vi "DG535.set input impedance.vi"(0 "i ref in":refnum<vi>, 7 "input impedance":bool, 11 "error in (no error)":errorcluster) -> (4 "i ref out":refnum<vi>, 15 "error out":errorcluster)   [LabVIEW 2014, in "DG535.lvlib"]
doc: "2 to 32766.\nThis command is used to specify the number of pulses, which will be in each burst of pulses when in the burst mode."
uses:
  DG535.lvlib
panel:
  # "50 Ohms"
  # "High Z"
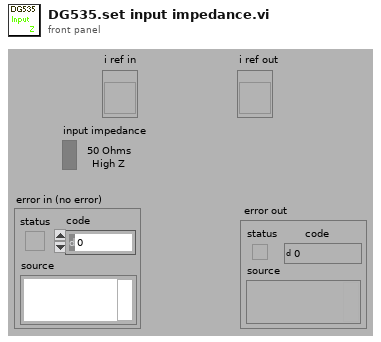
[diagram p1: front panel]
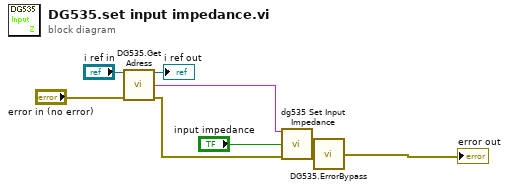
[diagram p0: block diagram]
diagram:
  n1 = call "DG535.Get Adress.vi"("i ref in"="i ref in", "error in (no error)"="error in (no error)") -> ("i ref out"=→"i ref out":refnum<vi>, "address"=w8:string, "error out"=w7:errorcluster)  [unwired: 10 in, 1 out]
  n2 = call "dg535 Set Input Impedance.vi"("address string"=w8, "input impedance"="input impedance", "error in"=w7) -> ("error out"=w6:errorcluster)  [unwired: 12 in]
  n3 = call "DG535.ErrorBypass.vi"("error in (no error)"=w6) -> ("error out"=→"error out":errorcluster)  [unwired: 14 in]
